vi "Detect Peak.vi"(4 "Num Samples":dbl=1000.0, 6 "Rate":dbl=10000.0, 8 "error in (no error)":errorcluster, 10 "Threshold":dbl=0.001, 11 "Filtered Signal":dynamicdata(waveform)) -> (0 "error out":errorcluster, 1 "Peak Amplitude":dbl, 2 "Peak Time Stamp":timestamp, 3 "Peak Found?":bool)   [LabVIEW 2020]
doc: "The Detect Peak VI takes the current <b>Num Samples</b> of <b>Filtered Signal</b> that was created at a specific <b>Rate</B> and determines if a peak was found above <b>Threshold</b>.\n\nIf a peak is found in the segment of data the <b>Peak Time Stamp</b> is returned in addition to the <b>Peak Amplitude</b>"
uses:
  <vilib>/Analysis/NI_AAL_SigProc.lvlib
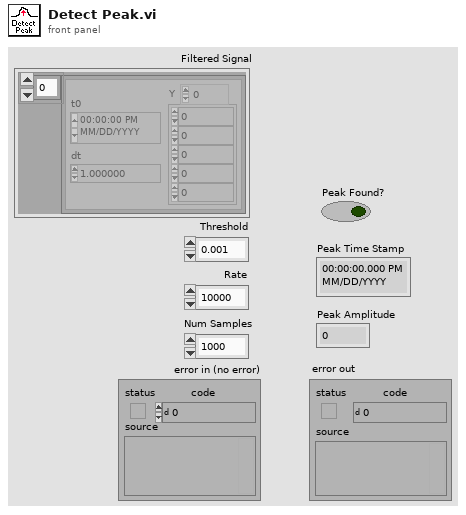
[diagram p1: front panel]
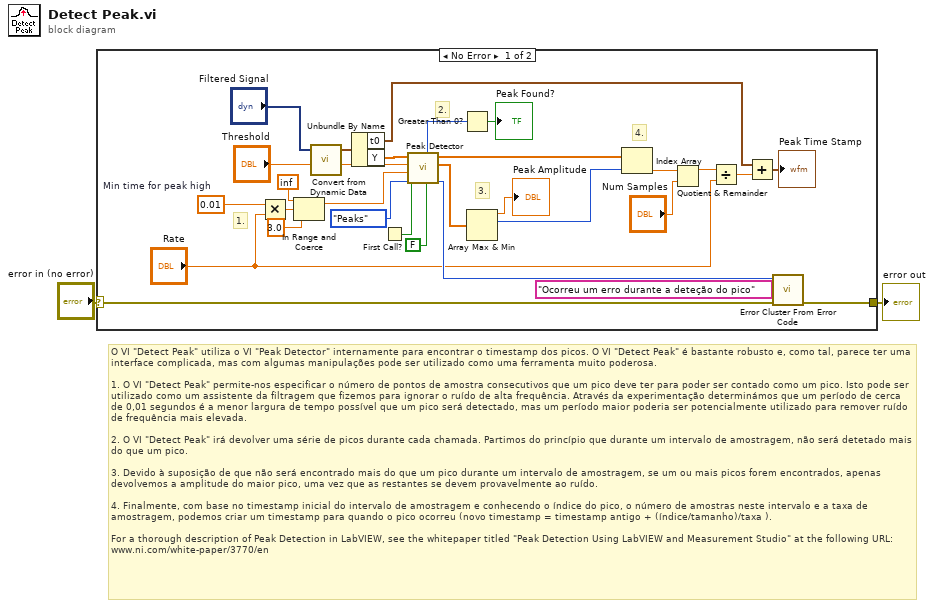
[diagram p0: block diagram]
diagram:
  # "O VI \"Detect Peak\" utiliza o VI \"Peak Detector\" internamente para encontrar o timestamp dos picos. O VI \"Detect Peak\" é bastante robusto e, como tal, parece ter uma interface complicada, mas com algumas manipulações pode ser utilizado como uma ferramenta muito poderosa.\n\n1. O VI \"Detect Peak\" permite-nos especificar o número de pontos de amostra consecutivos que um pico deve ter para poder ser contado como um pico. Isto pode ser utilizado como um assistente da filtragem que fizemos para ignorar o ruído de alta frequência. Através da experimentação determinámos que um período de cerca de 0,01 segundos é a menor largura de tempo possível que um pico será detectado, mas um período maior poderia ser potencialmente utilizado para remover ruído de frequência mais elevada.\n\n2. O VI \"Detect Peak\" irá devolver uma série de picos durante cada chamada. Partimos do princípio que durante um intervalo de amostragem, não será detetado mais do que um pico.\n\n3. Devido à suposição de que não será encontrado mais do que um pico durante um intervalo de amostragem, se um ou mais picos forem encontrados, apenas devolvemos a amplitude do maior pico, uma vez que as restantes se devem provavelmente ao ruído.\n\n4. Finalmente, com base no timestamp inicial do intervalo de amostragem e conhecendo o índice do pico, o número de amostras neste intervalo e a taxa de amostragem, podemos criar um timestamp para quando o pico ocorreu (novo timestamp = timestamp antigo + (índice/tamanho)/taxa ).\n\nFor a thorough description of Peak Detection in LabVIEW, see the whitepaper titled \"Peak Detection Using LabVIEW and Measurement Studio\" at the following URL:  www.ni.com/white-paper/3770/en"
  n1 = case shown="No Error" "error in (no error)" {
    selector: "error in (no error)" -> [w16 w32]
    tunnel: [w13 w32] -> w1
    frame No Error {
      w11 = 0.01  # Min time for peak high
      # "4."
      # "3."
      # "2."
      # "1."
      n2 = Multiply(x=w11, y="Rate") -> (x*y=w6:dbl)
      n3 = In Range and Coerce(upper limit=inf, x=w6, lower limit=3.0) -> (coerced(x)=w5:dbl)  [unwired: 1 out]
      n4 = call "Convert from Dynamic Data"("Dynamic Data Type"="Filtered Signal") -> ("Waveform"=w29:waveform(dbl))  [unwired: 3 in]
      n5 = Unbundle By Name(w29) -> ("t0"=w19:timestamp, "Y"=w31:dbl[])
      n6 = First Call?() -> (First Call?: T/F=w27:bool)
      n7 = call <vilib>:"Peak Detector.vi"("end of data (T)"=FALSE, "initialize (T)"=w27, "peaks/valleys"=enum32{"Peaks", "Valleys"}."Peaks", "width"=w5, "threshold"="Threshold", "X"=w31) -> ("error"=w15:i32, "Amplitudes"=w9:dbl[], "Locations"=w28:dbl[], "# found"=w10:i32)  [unwired: 1 in, 1 out]
      n8 = Greater Than 0?(x=w10) -> (x > 0?=→"Peak Found?":bool)
      n9 = Array Max & Min(array=w9) -> (max value=→"Peak Amplitude":dbl, max index (indices)=w8:i32)  [unwired: 2 out]
      n10 = Index Array(array=w28, index=w8) -> (element=w18:dbl)
      n11 = Quotient & Remainder(x=w18, y="Num Samples") -> (x-y*floor(x/y)=w20:dbl)  [unwired: 1 out]
      n12 = Divide(x=w20, y="Rate") -> (x/y=w22:dbl)
      n13 = Add(x=w19, y=w22) -> (x+y=→"Peak Time Stamp":timestamp)
      n14 = call <vilib>:"Error Cluster From Error Code.vi"("error in (no error)"=w16, "error message (\"\")"="Ocorreu um erro durante a deteção do pico" ("error message (\"\")"), "error code (0)"=w15) -> ("error out"=w13:errorcluster)  [unwired: 6 in]
    }
    frame Error {
    }
  }
  "error out" <- w1
